vi "Facade 1.vi"(0 "Data In":T4, 2 "Display State In":T2, 3 "Container State":T3) -> (6 "Data Out":T4, 7 "Display State Out":T2, 8 "Action":T1)   [LabVIEW 2012, in "Custom Combo Box.xctl"]
uses:
  Custom Combo Box.xctl
  Data 1.ctl
  <vilib>/_xctls/Container State.ctl
  State 1.ctl
  <vilib>/_xctls/Action.ctl
  <vilib>/_xctls/XControlSupport.lvlib
panel:
  in  "Combo Box":string(combo)
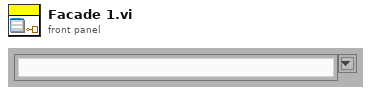
[diagram p1: front panel]
types:
  T1 = typedef "XControlSupport.lvlib/Action.ctl" = cluster{"Data Changed?":bool, "State Changed?":bool, "Action Name":string}
  T2 = typedef "Custom Combo Box.xctl/State 1.ctl" = cluster{"String":string}
  T3 = typedef "XControlSupport.lvlib/Container State.ctl" = cluster{"Indicator?":bool, "Run Mode?":bool, " Refnum":refnum<vi>}
  T4 = typedef "Custom Combo Box.xctl/Data 1.ctl" = cluster{"String":string, "Value":string}[]
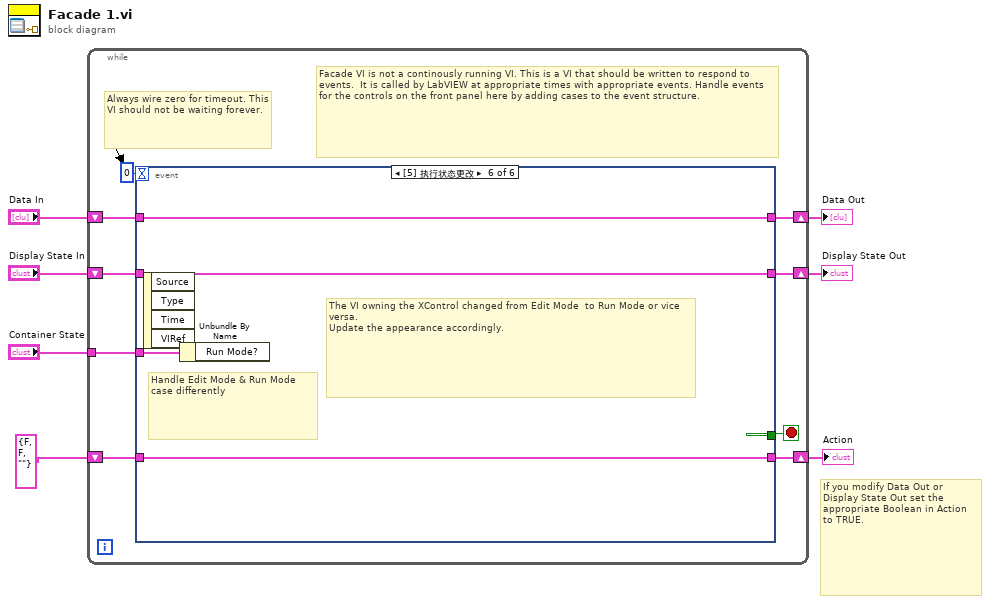
[diagram p0: block diagram]
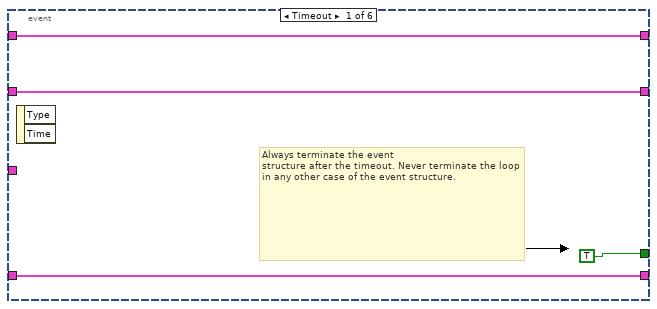
[diagram p2: hidden frame]
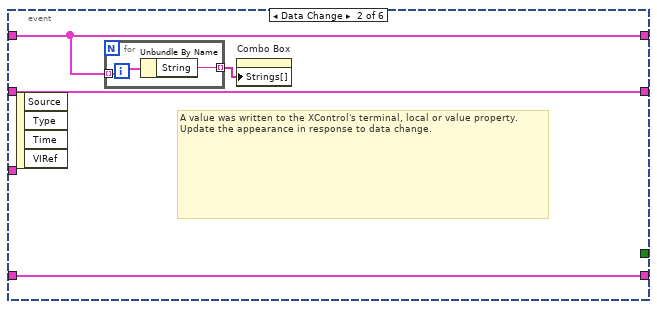
[diagram p3: hidden frame]
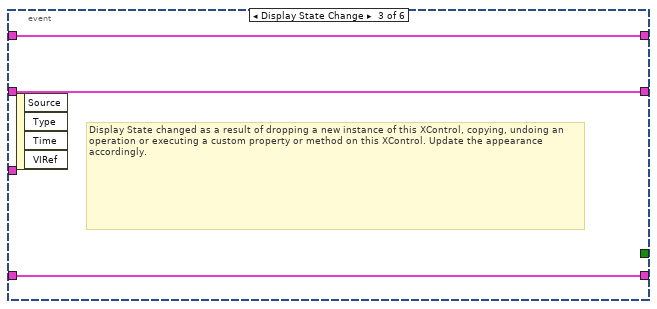
[diagram p4: hidden frame]
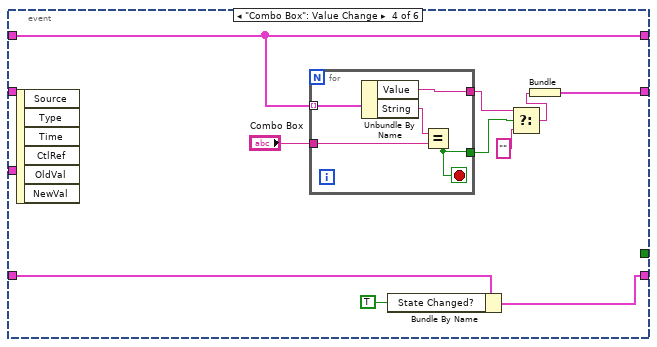
[diagram p5: hidden frame]
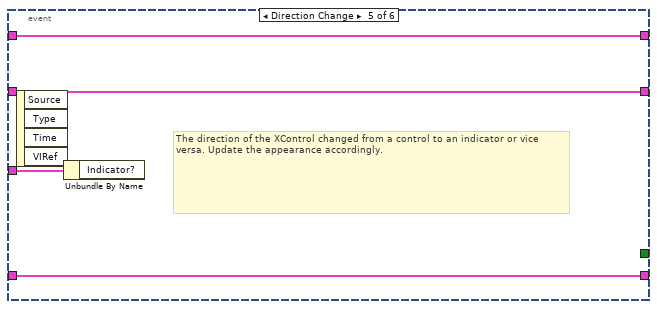
[diagram p6: hidden frame]
diagram:
  # "If you modify Data Out or\nDisplay State Out set the\nappropriate Boolean in Action\nto TRUE."
  n1 = while {
    shift-right: [w15] -> w4
    shift-left: "Display State In" -> [w16]
    tunnel: "Container State" -> [w12]
    shift-right: [w10] -> w7
    shift-left: "Data In" -> [w11]
    shift-right: [w8] -> w2
    shift-left: T1 {"Data Changed?"=FALSE, "State Changed?"=FALSE, "Action Name"=""} ("Action") -> [w9]
    stop <- w14 stop-if-true
    # "Facade VI is not a continously running VI. This is a VI that should be written to respond to events.  It is called by LabVIEW at appropriate times with appropriate events. Handle events for the controls on the front panel here by adding cases to the event structure."
    # "Always wire zero for timeout. This\nVI should not be waiting forever."
    n2 = event shown="[5] 执行状态更改" {
      selector: _ -> [_ _ _ _ _ _]
      dyn-events: _ -> [_ _ _ _ _ _]
      timeout: 0 -> [_ _ _ _ _ _]
      tunnel: w16 -> [w18 w24 w29 _ w47 w51]
      tunnel: [w18 w24 w29 w37 w47 w51] -> w15
      tunnel: [TRUE _ _ _ _ _] -> w14
      tunnel: w12 -> [_ _ _ _ w48 w52]
      tunnel: w11 -> [w17 w21 w28 w39 w46 w49]
      tunnel: [w17 w21 w28 w39 w46 w49] -> w10
      tunnel: [w19 w23 w27 w34 w45 w50] -> w8
      tunnel: w9 -> [w19 w23 w27 w36 w45 w50]
      event Timeout {
        # "Always terminate the event\nstructure after the timeout. Never terminate the loop in any other case of the event structure."
        n3 = event-data() -> ()  [unwired: 3 out]
      }
      event Data Change {
        # "A value was written to the XControl's terminal, local or value property.\nUpdate the appearance in response to data change."
        n4 = event-data() -> ()  [unwired: 5 out]
        n5 = for {
          tunnel: w21 -> [w26] mode=indexing
          tunnel: [w25] -> w22 mode=indexing
          n6 = Unbundle By Name(w26) -> ("String"=w25:string)
        }
        n7 = property on="Combo Box" class="CmbBox"("Strings[]"=w22) -> ()  [unwired: 2 in, 2 out]
      }
      event Display State Change {
        # "Display State changed as a result of dropping a new instance of this XControl, copying, undoing an operation or executing a custom property or method on this XControl. Update the appearance accordingly."
        n8 = event-data() -> ()  [unwired: 5 out]
      }
      event "Combo Box": Value Change {
        n9 = event-data() -> ()  [unwired: 7 out]
        n10 = for {
          tunnel: w39 -> [w44] mode=indexing
          tunnel: "Combo Box" -> [w43]
          tunnel: [w41] -> w32
          tunnel: [w40] -> w33
          stop <- w40 stop-if-true
          n11 = Unbundle By Name(w44) -> ("Value"=w41:string, "String"=w42:string)
          n12 = Equal?(x=w42, y=w43) -> (x = y?=w40:bool)
        }
        n13 = Bundle By Name(cluster=w36, "State Changed?"=TRUE) -> (w34:T1)
        n14 = Select(t=w32, s=w33, f="") -> (s? t:f=w31:string)
        n15 = Bundle("f"=w31) -> (w37:cluster{"f":string})  [unwired: 1 in]
      }
      event Direction Change {
        # "The direction of the XControl changed from a control to an indicator or vice versa. Update the appearance accordingly."
        n16 = event-data() -> ()  [unwired: 5 out]
        n17 = Unbundle By Name(w48) -> ()  [unwired: 1 out]
      }
      event Exec State Change {
        # "The VI owning the XControl changed from Edit Mode  to Run Mode or vice versa.\nUpdate the appearance accordingly."
        # "Handle Edit Mode & Run Mode\ncase differently"
        n18 = event-data() -> ()  [unwired: 5 out]
        n19 = Unbundle By Name(w52) -> ()  [unwired: 1 out]
      }
    }
  }
  "Display State Out" <- w4
  "Data Out" <- w7
  "Action" <- w2
